vi "MoveTo.vi"(4 "Curr Pos":dbl, 5 "Desired Pos":dbl, 7 "Axis Name":string, 10 "Steps/unit":dbl) -> (2 "Anything move?":bool)   [LabVIEW 2015]
panel:
  out "Numeric":dbl
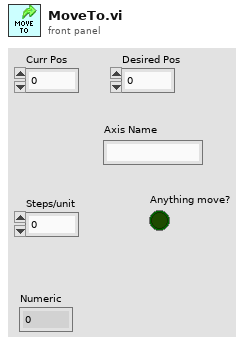
[diagram p1: front panel]
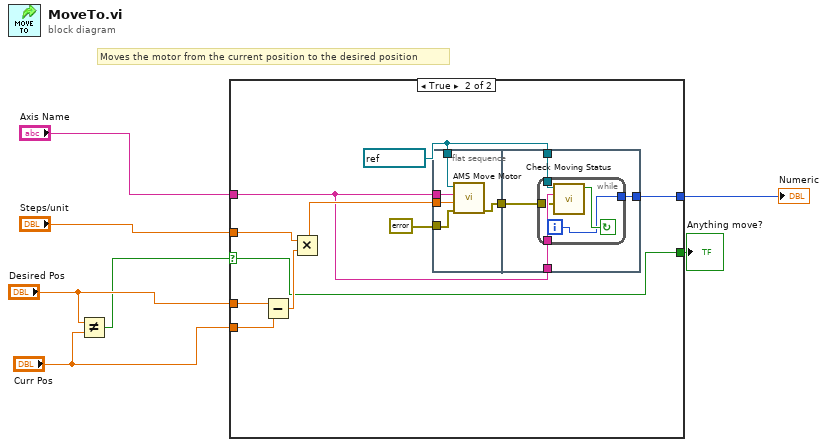
[diagram p0: block diagram]
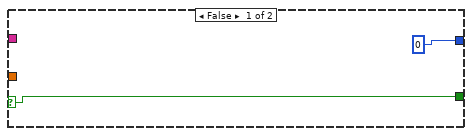
[diagram p2: hidden frame]
diagram:
  # "Moves the motor from the current position to the desired position"
  n1 = Not Equal?(x="Desired Pos", y="Curr Pos") -> (x != y?=w3:bool)
  n2 = case shown="True" w3 {
    selector: w3 -> [w9 w14]
    tunnel: "Desired Pos" -> [_ w20]
    tunnel: "Steps/unit" -> [_ w19]
    tunnel: "Axis Name" -> [_ w12]
    tunnel: "Curr Pos" -> [_ w18]
    tunnel: [w9 w14] -> w2
    tunnel: [0 w10] -> w1
    frame False {
    }
    frame True {
      w13 = refnum<visa-resource-name> "COM5" ("VISA resource name IN")
      n3 = Subtract(x=w20, y=w18) -> (x-y=w17:dbl)
      n4 = Multiply(x=w19, y=w17) -> (x*y=w16:dbl)
      n5 = flat-sequence {
        tunnel: w12 -> [w25]
        tunnel: w13 -> [w24]
        tunnel: w16 -> [w23]
        tunnel: errorcluster {"status"=FALSE, "code"=0, "source"=""} ("error constant") -> [w22]
        tunnel: [w21] -> w11
        tunnel: w13 -> [w29]
        tunnel: w12 -> [w28]
        tunnel: w11 -> [w27]
        tunnel: [w26] -> w10
        frame #0 {
          n6 = call "AMS Move Motor.vi"("error in"=w22, "Motor steps"=w23, "Axis Prefix"=w25, "VISA resource name IN"=w24) -> ("error out"=w21:errorcluster)  [unwired: 6 in, 1 out]
        }
        frame #1 {
          n7 = while {
            tunnel: w29 -> [w34]
            tunnel: w28 -> [w33]
            tunnel: w27 -> [w32]
            tunnel: [w30] -> w26
            i -> [w30]
            stop <- w31 continue-if-true
            n8 = call "Check Moving Status.vi"("error in (no error)"=w32, "Axis Prefix"=w33, "VISA Refnum in"=w34) -> ("Moving?"=w31:bool)  [unwired: 6 in, 2 out]
          }
        }
      }
    }
  }
  "Anything move?" <- w2
  "Numeric" <- w1
